vi "example_boolUserEventStopMechanism.vi"() -> ()   [LabVIEW 2023]
doc: "This example demonstrates the use of TLC_Daemon for launching, controlling, and stopping asynchronous background tasks in a clean, object-oriented manner. It utilizes a boolean user event mechanism to stop active tasks."
uses:
  TaskController/TaskController.lvclass
  Task_BoolUserEventStopMech/Task_BoolUserEventStopMech.lvclass
panel:
  out "error":errorcluster
  in  "stop":bool
  in  "launchNewTask":bool
  # "Example of TaskController with Boolean User Event Stop Mechanism"
  # "Instruction:\n1. Press RUN button.\n\n2. Press LAUNCH NEW TASK button to launch a new task \n\n3. Press STOP button to stop all the active tasks using the Boolean User Event Stop Mechanism\n\nFor details, view code and its comments"
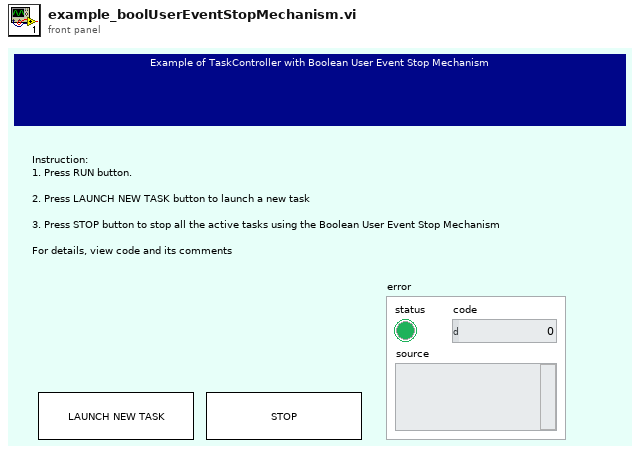
[diagram p1: front panel]
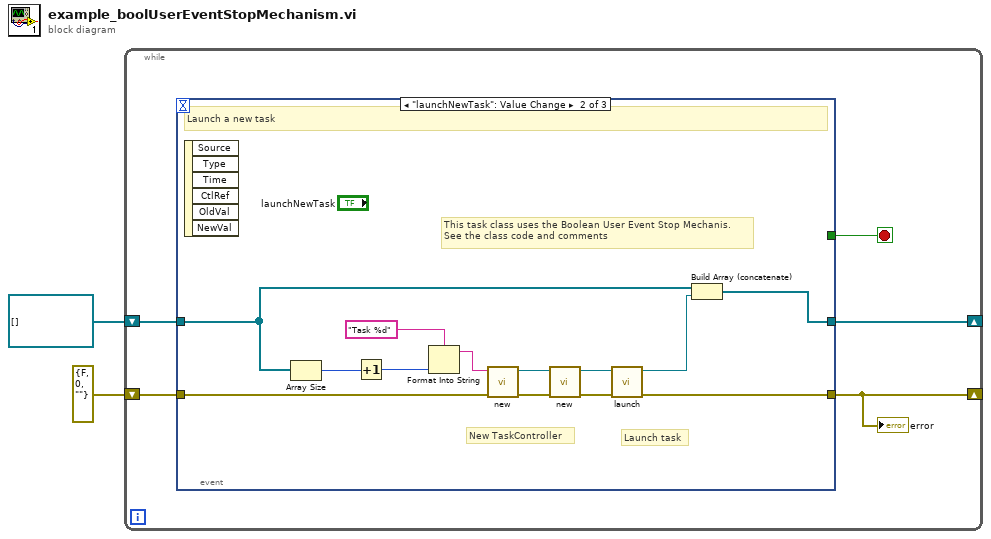
[diagram p0: block diagram]
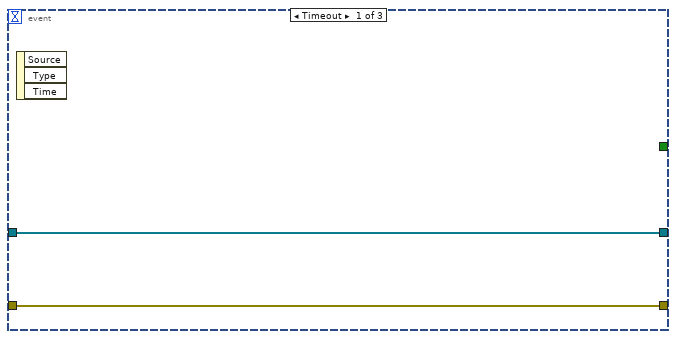
[diagram p2: hidden frame]
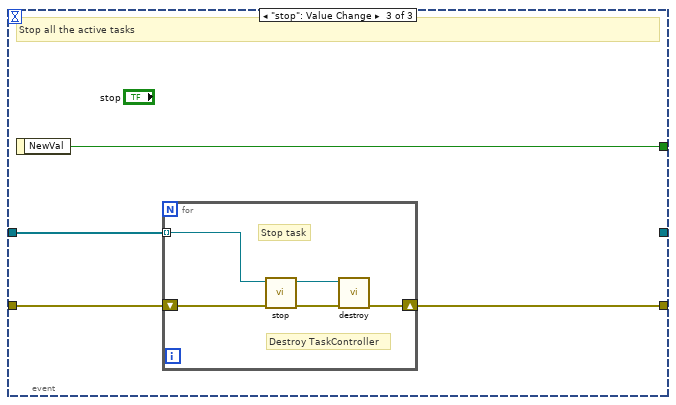
[diagram p3: hidden frame]
diagram:
  n1 = while {
    shift-right: [w7] -> _
    shift-left: refnum<class "TaskController.lvclass">[] [] -> [w6]
    shift-right: [w3] -> _
    shift-left: errorcluster {"status"=FALSE, "code"=0, "source"=""} -> [w5]
    stop <- w4 stop-if-true
    n2 = event shown="[1] \"launchNewTask\": Value Change" {
      selector: _ -> [_ _ _]
      dyn-events: _ -> [_ _ _]
      timeout: _ -> [_ _ _]
      tunnel: [w9 w17 _] -> w7
      tunnel: w6 -> [w9 w14 w26]
      tunnel: [w8 w16 w24] -> w3
      tunnel: w5 -> [w8 w15 w25]
      tunnel: [_ _ w23] -> w4
      event Timeout {
        n3 = event-data() -> ()  [unwired: 1 in, 3 out]
      }
      event "launchNewTask": Value Change {
        # "This task class uses the Boolean User Event Stop Mechanis.\nSee the class code and comments"
        # "New TaskController"
        # "Launch task"
        # "Launch a new task"
        n4 = event-data() -> ()  [unwired: 1 in, 6 out]
        n5 = Array Size(array=w14) -> (size(s)=w11:i32)
        n6 = Increment(x=w11) -> (x+1=w13:i32)
        n7 = Format Into String(format string="Task %d", w13) -> (resulting string=w10:string)  [unwired: 2 in, 1 out]
        n8 = call "new.vi"("error in (no error)"=w15, "description"=w10) -> ("error out"=w22:errorcluster, "ExampleTask_StopNotifier out"=w19:refnum<class "Task_BoolUserEventStopMech.lvclass">)  [unwired: 8 in]
        n9 = call "new.vi"("error in (no error)"=w22, "task"=w19) -> ("error out"=w21:errorcluster, "TaskController out"=w20:refnum<class "TaskController.lvclass">)  [unwired: 8 in]
        n10 = call "launch.vi"("error in (no error)"=w21, "TaskController in"=w20) -> ("error out"=w16:errorcluster, "TaskController out"=w18:refnum<class "TaskController.lvclass">)  [unwired: 8 in]
        n11 = Build Array (concatenate)(w14, w18) -> (w17:refnum<class "TaskController.lvclass">[])
      }
      event "stop": Value Change {
        # "Stop all the active tasks"
        n12 = event-data() -> ("NewVal"=w23:bool)  [unwired: 1 in]
        n13 = for {
          tunnel: w26 -> [w29] mode=indexing
          shift-right: [w27] -> w24
          shift-left: w25 -> [w28]
          # "Destroy TaskController"
          # "Stop task"
          n14 = call "stop.vi"("error in (no error)"=w28, "TaskController in"=w29) -> ("error out"=w30:errorcluster, "TaskController out"=w31:refnum<class "TaskController.lvclass">)  [unwired: 8 in]
          n15 = call "destroy.vi"("error in (no error)"=w30, "TaskController in"=w31) -> ("error out"=w27:errorcluster)  [unwired: 7 in, 2 out]
        }
      }
    }
    "error" <- w3
  }
